vi "Create.vi"(8 "error in (no error)":errorcluster, 9 "LoggerName":string, 10 "SubPanelRef":refnum<vi>) -> (0 "error out":errorcluster, 3 "ConsoleOutput out":refnum<class "ConsoleOutput.lvclass">)   [LabVIEW 2020, in "ConsoleOutput.lvclass"]
uses:
  ConsoleOutput.lvclass
  Lib/HSE-Logger/LogLevel.ctl
  Private/TypeDef/LogEventsRefum.ctl
  Lib/HSE-Logger/LogRecord/LogRecord.lvclass
  ConsoleOutput.lvclass/ConsoleOutput.ctl
  Lib/HSE-Logger/Handler/UserEventHandler/UserEventHandler.lvclass
  E:/My-LV-OOP-Design-Patterns/SupportLibs/HSE-Logger/Handler/Handler.lvclass
  Lib/hse-logger.lvlib
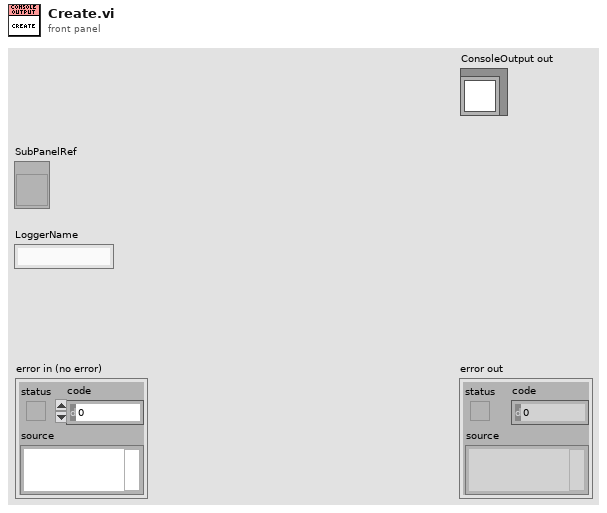
[diagram p1: front panel]
types:
  T1 = typedef "hse-logger.lvlib/LogLevel.ctl" = enum16{"DEBUG", "INFO", "WARNING", "ERROR", "CRITICAL"}
  T2 = typedef "ConsoleOutput.lvclass/LogEventsRefum.ctl" = cluster{"LogRecord":refnum<user-event>, "Stop":refnum<user-event>}
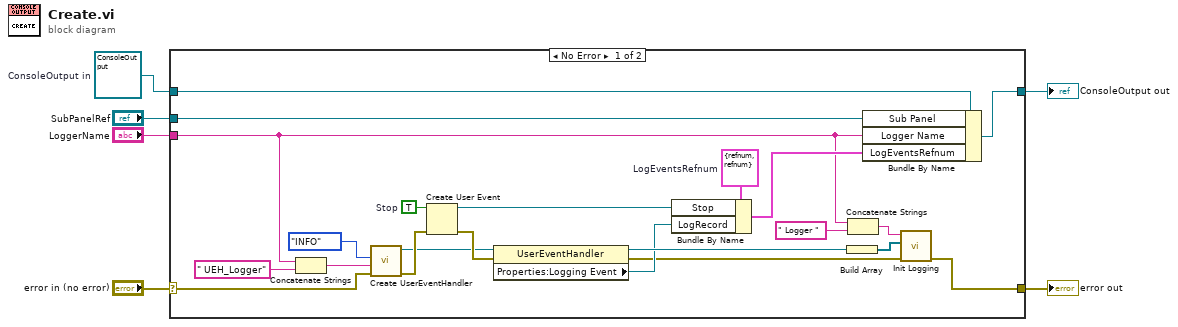
[diagram p0: block diagram]
diagram:
  w1 = refnum<class "ConsoleOutput.lvclass"> refnum  # ConsoleOutput in
  n1 = case shown="No Error" "error in (no error)" {
    selector: "error in (no error)" -> [w25 w30]
    tunnel: [w24 w30] -> w5
    tunnel: [w18 w29] -> w4
    tunnel: "LoggerName" -> [w14 _]
    tunnel: "SubPanelRef" -> [w19 _]
    tunnel: w1 -> [w7 w29]
    frame No Error {
      w16 = T2 {"LogRecord"=refnum, "Stop"=refnum}  # LogEventsRefnum
      w17 = TRUE  # Stop
      n2 = Concatenate Strings(w14, " UEH_Logger" ("Name")) -> (w22:string)
      n3 = call "Create UserEventHandler.vi"("error in"=w25, "Name"=w22, "Level"=LogLevel."INFO") -> ("error out"=w13:errorcluster, "UserEventHandler out"=w11:refnum<class "UserEventHandler.lvclass">)  [unwired: 7 in]
      n4 = Create User Event(user event datatype=w17, error in=w13) -> (user event=w10:refnum<user-event>, error out=w12:errorcluster)
      n5 = property class="UserEventHandler"(reference=w11, error in=w12) -> (reference out=w27:refnum<class "UserEventHandler.lvclass">, error out=w8:errorcluster, "Properties:Logging Event"=w9:refnum<user-event>)
      n6 = Bundle By Name(cluster=w16, "Stop"=w10, "LogRecord"=w9) -> (w15:T2)
      n7 = Build Array(w27) -> (w28:refnum<class "UserEventHandler.lvclass">[])
      n8 = Concatenate Strings(w14, " Logger " ("Name")) -> (w20:string)
      n9 = Bundle By Name(cluster=w7, "Sub Panel"=w19, "Logger Name"=w14, "LogEventsRefnum"=w15) -> (w18:refnum<class "ConsoleOutput.lvclass">)
      n10 = call "Init Logging.vi"("error in"=w8, "Handlers"=w28, "Name"=w20) -> ("error out"=w24:errorcluster)  [unwired: 8 in]
    }
    frame Error {
    }
  }
  "error out" <- w5
  "ConsoleOutput out" <- w4
